vi "Minesweeper.vi"() -> ()   [LabVIEW 2018]
uses:
  ecc87c49-68d8-480b-962c-e2d9a9991d5a.vi
panel:
  in  "I did not survive and \nneed to try again:(":bool
  in  "Array":bool[][](array[boolean])
  out "Array 2":picture[][](array[picture])
  # "MINESWEEPER"
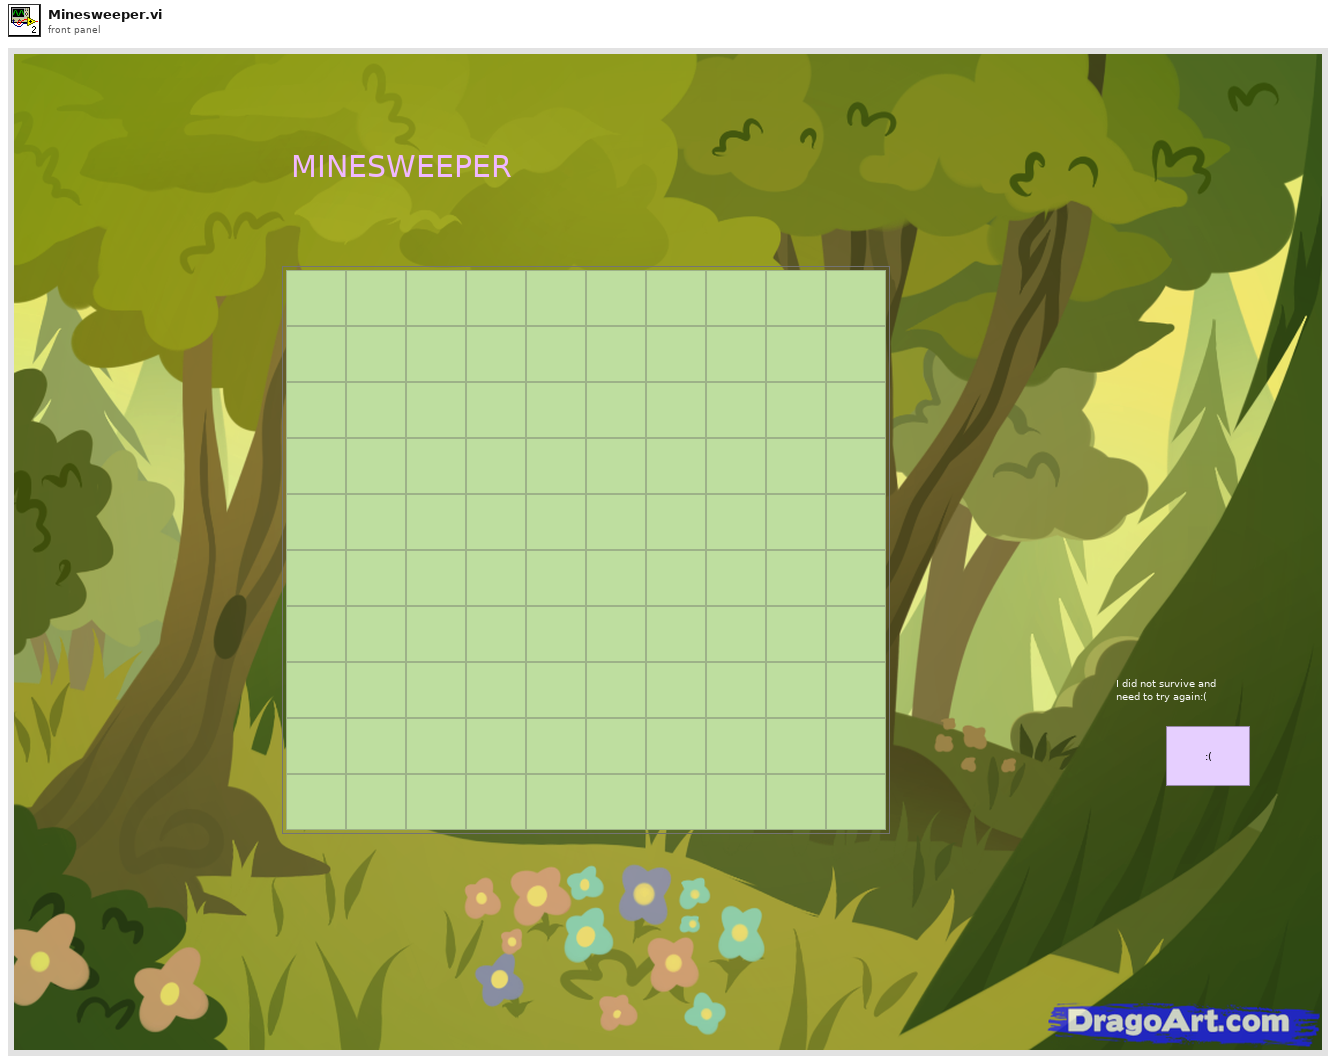
[diagram p1: front panel]
types:
  T1 = enum16{"Initialize", "Wait for event", "Game", "Analyze", "User msg", "New", "End"}
  T2 = typedef "imagedata.ctl" = cluster{"image type":i32, "image depth":i32, "image":u8[], "mask":u8[], "colors":u32[], "Rectangle":cluster{"left":i16, "top":i16, "right":i16, "bottom":i16}}
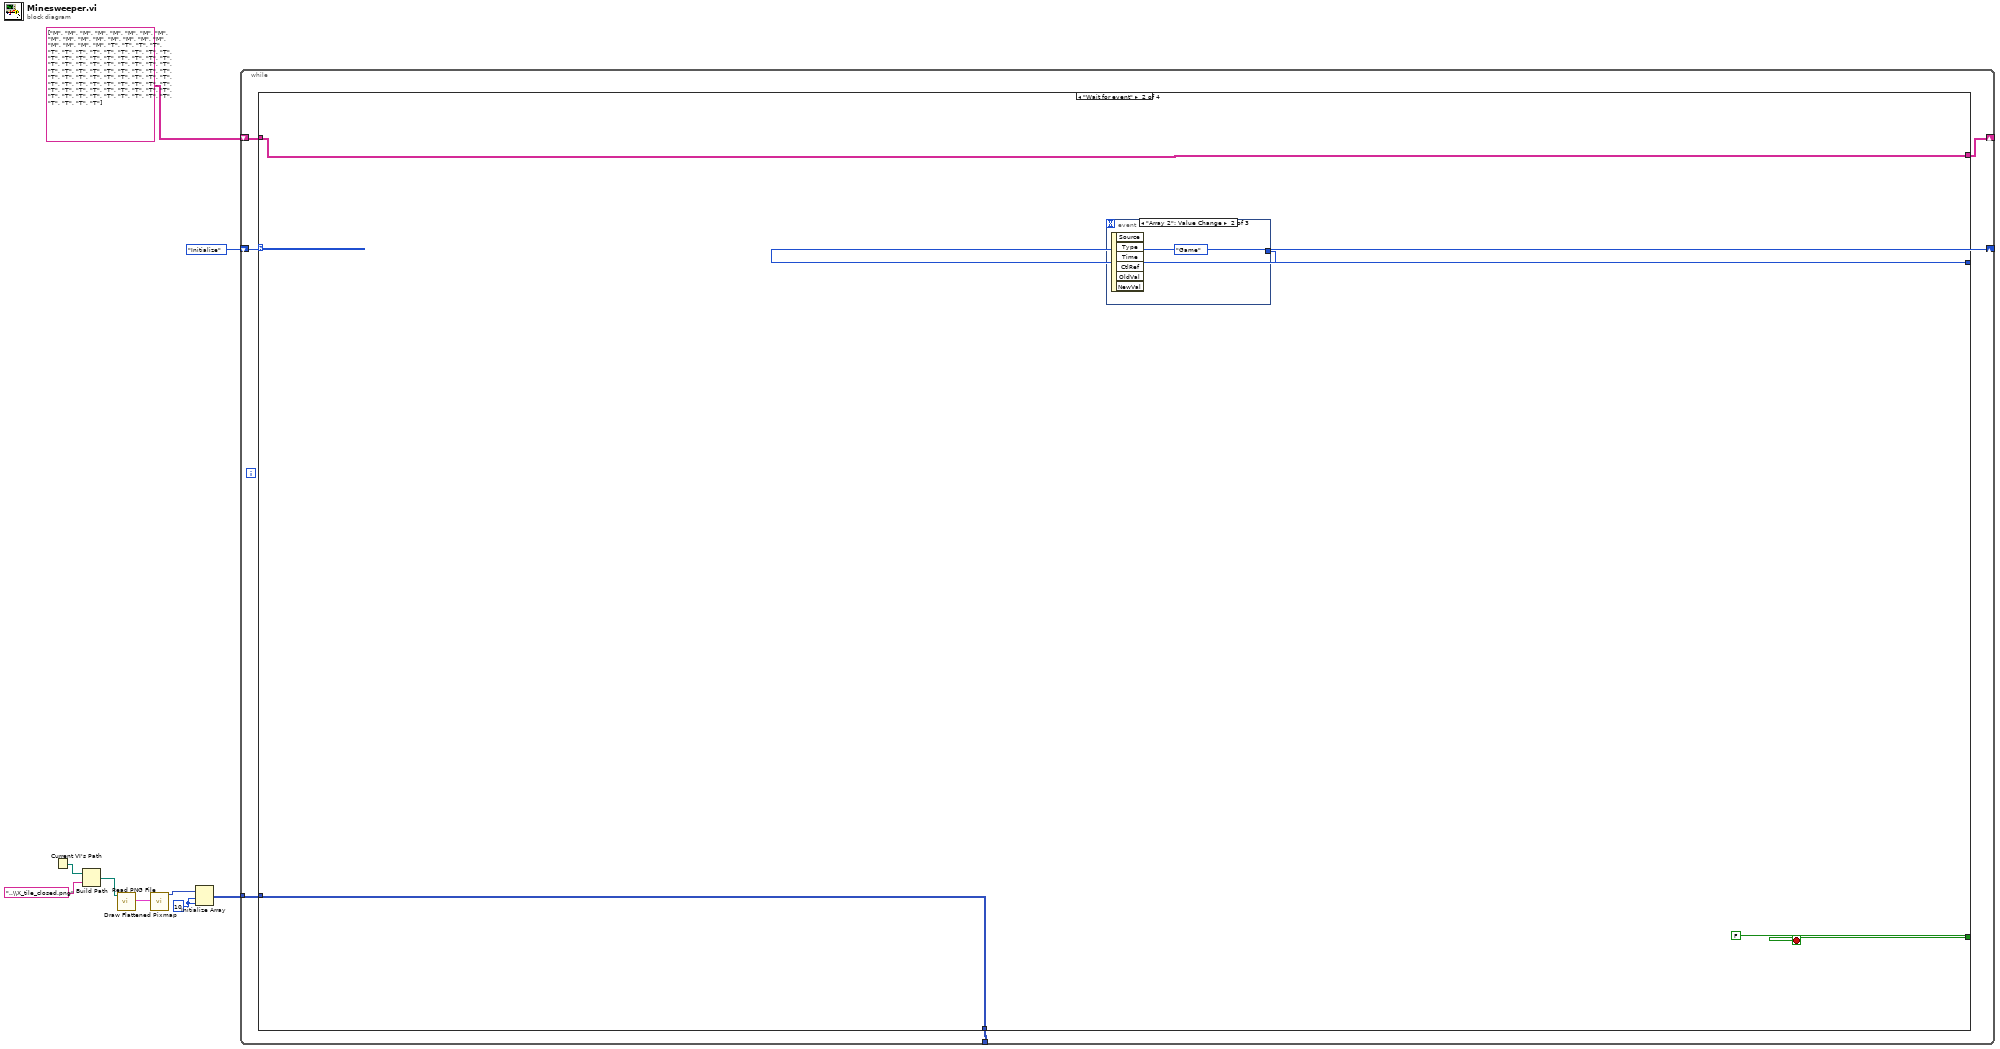
[diagram p0: block diagram]
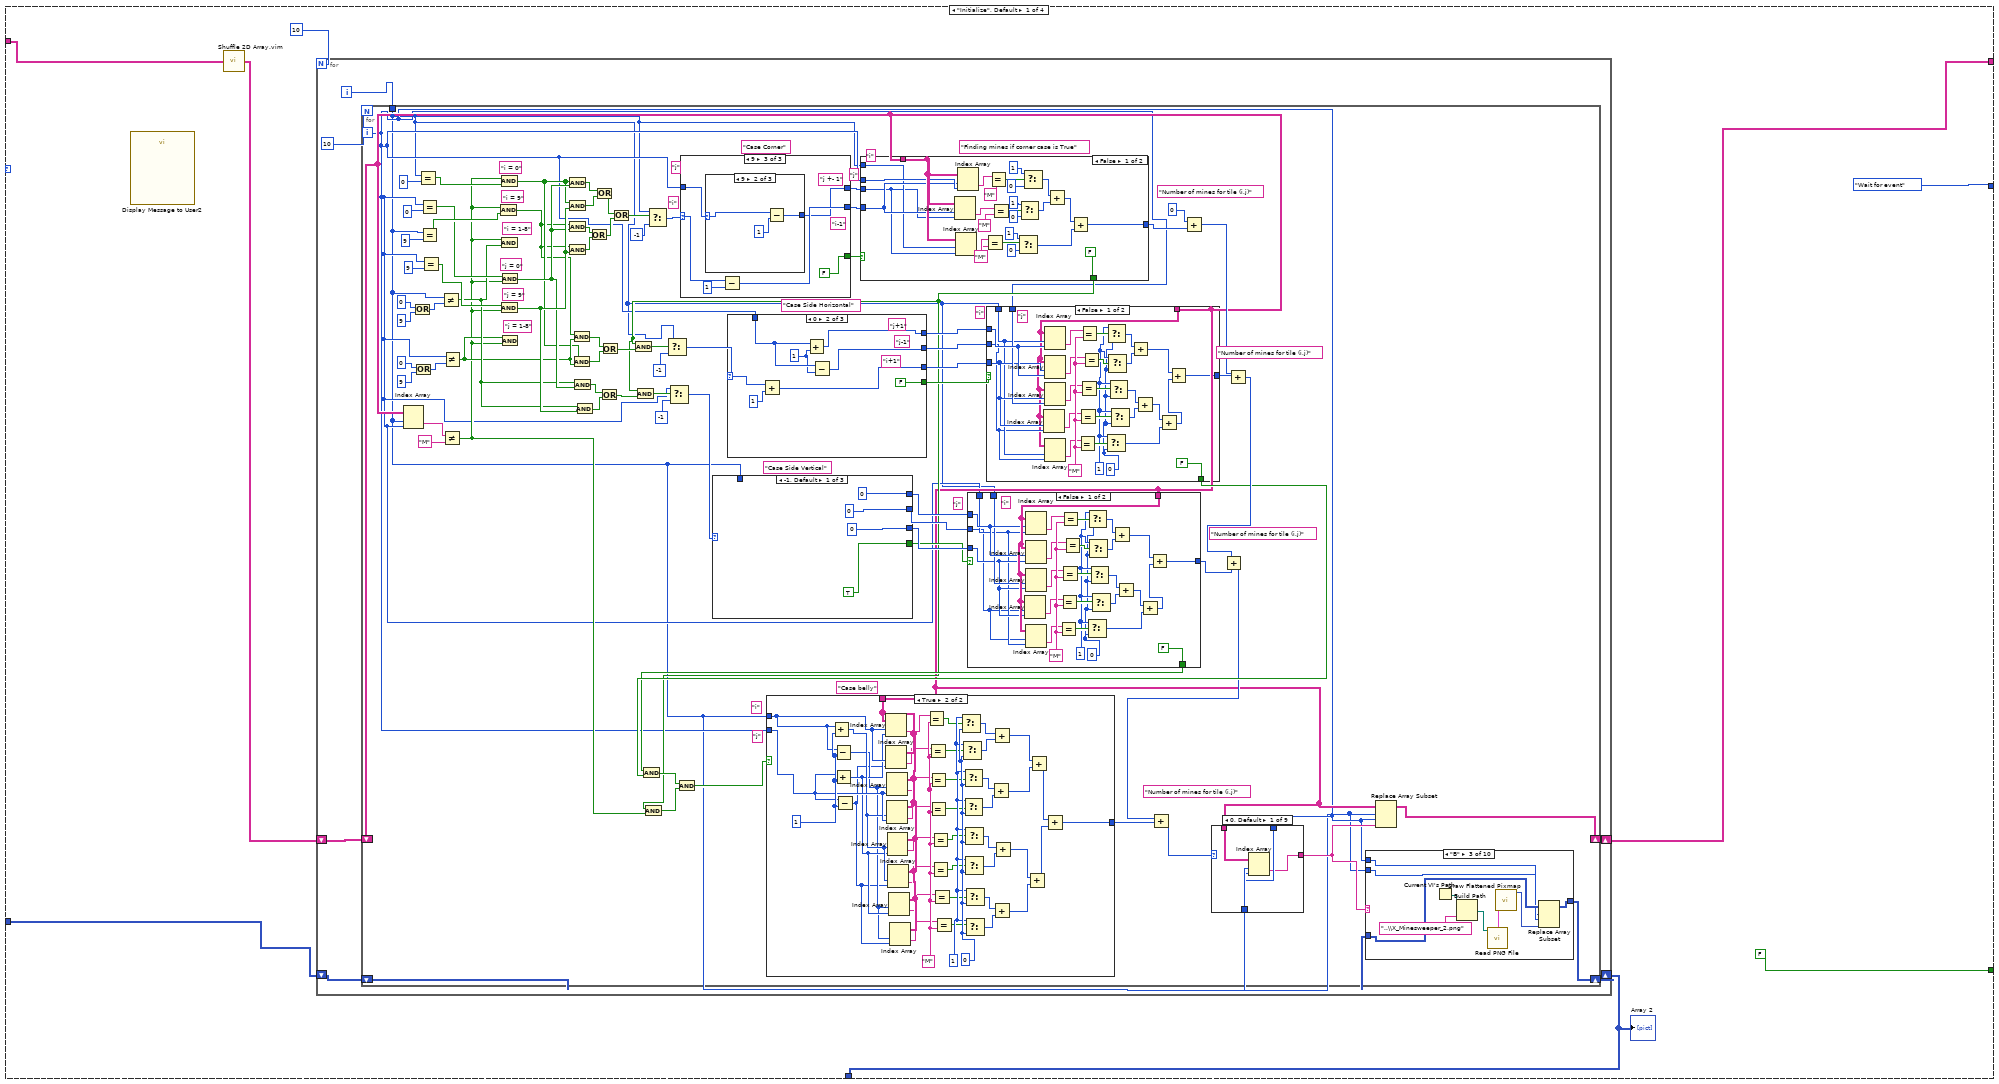
[diagram p2: hidden frame]
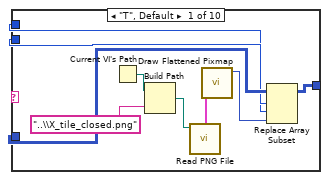
[diagram p3: hidden frame]
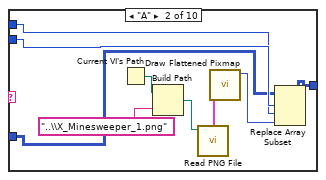
[diagram p4: hidden frame]
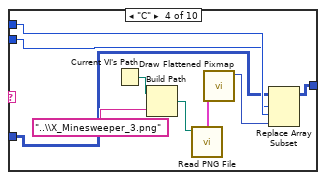
[diagram p5: hidden frame]
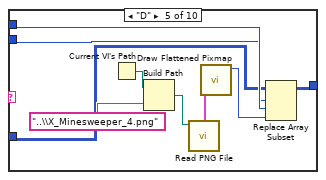
[diagram p6: hidden frame]
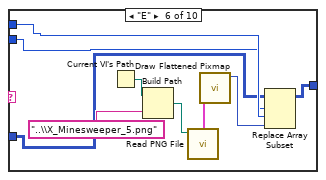
[diagram p7: hidden frame]
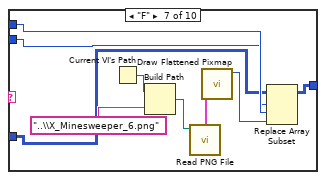
[diagram p8: hidden frame]
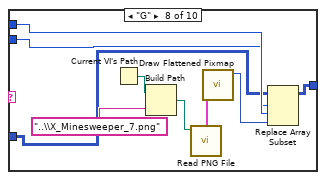
[diagram p9: hidden frame]
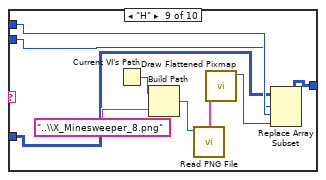
[diagram p10: hidden frame]
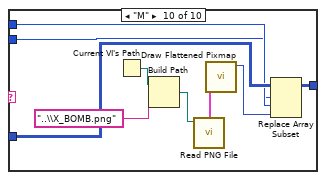
[diagram p11: hidden frame]
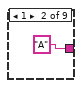
[diagram p12: hidden frame]
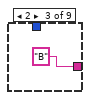
[diagram p13: hidden frame]
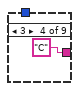
[diagram p14: hidden frame]
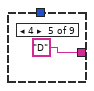
[diagram p15: hidden frame]
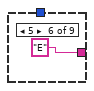
[diagram p16: hidden frame]
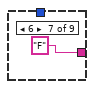
[diagram p17: hidden frame]
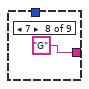
[diagram p18: hidden frame]
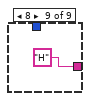
[diagram p19: hidden frame]
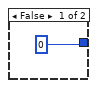
[diagram p20: hidden frame]
diagram:
  w2 = 10
  n1 = Current VI's Path() -> (path=w4:path)
  n2 = Build Path(base path=w4, name or relative path="..\\X_tile_closed.png") -> (appended path=w5:path)
  n3 = call <vilib>:"Read PNG File.vi"("path to PNG file"=w5) -> ("image data"=w6:T2)  [unwired: 8 in, 2 out]
  n4 = call <vilib>:"Draw Flattened Pixmap.vi"("image data"=w6) -> ("new picture"=w7:picture)  [unwired: 8 in]
  n5 = Initialize Array(w7, w2, w2) -> (w1:picture[][])
  n6 = while {
    shift-right: [w15] -> _
    shift-left: T1."Initialize" -> [w16]
    tunnel: w1 -> [w13]
    tunnel: [w12] -> _
    shift-right: [w10] -> _
    shift-left: string[][] [["M", "M", "M", "M", "M", "M", "M", "M", "M", "M"], ["M", "M", "M", "M", "M", "M", "M", "M", "M", "M"], ["T", "T", "T", "T", "T", "T", "T", "T", "T", "T"], ["T", "T", "T", "T", "T", "T", "T", "T", "T", "T"], ["T", "T", "T", "T", "T", "T", "T", "T", "T", "T"], ["T", "T", "T", "T", "T", "T", "T", "T", "T", "T"], ["T", "T", "T", "T", "T", "T", "T", "T", "T", "T"], ["T", "T", "T", "T", "T", "T", "T", "T", "T", "T"], ["T", "T", "T", "T", "T", "T", "T", "T", "T", "T"], ["T", "T", "T", "T", "T", "T", "T", "T", "T", "T"]] -> [w11]
    stop <- w14 stop-if-true
    n7 = case shown="\"Wait for event\"" w16 {
      tunnel: [w20 w416 w429 string[][] [["M", "M", "M", "M", "M", "M", "M", "M", "M", "M"], ["M", "M", "M", "M", "M", "M", "M", "M", "M", "M"], ["T", "T", "T", "T", "T", "T", "T", "T", "T", "T"], ["T", "T", "T", "T", "T", "T", "T", "T", "T", "T"], ["T", "T", "T", "T", "T", "T", "T", "T", "T", "T"], ["T", "T", "T", "T", "T", "T", "T", "T", "T", "T"], ["T", "T", "T", "T", "T", "T", "T", "T", "T", "T"], ["T", "T", "T", "T", "T", "T", "T", "T", "T", "T"], ["T", "T", "T", "T", "T", "T", "T", "T", "T", "T"], ["T", "T", "T", "T", "T", "T", "T", "T", "T", "T"]]] -> w10
      tunnel: [T1."Wait for event" w417 T1."Wait for event" T1."Initialize"] -> w15
      tunnel: [FALSE FALSE FALSE FALSE] -> w14
      tunnel: [w19 w415 w427 w457] -> w12
      tunnel: w13 -> [w18 w415 w427 w457]
      tunnel: w11 -> [w17 w416 w429 _]
      frame "Initialize", Default {
        n8 = call "Display Message to User2"() -> ()  [unwired: 10 in, 2 out]
        n9 = call "Shuffle 2D Array.vim"("array"=w17) -> ("shuffled array"=w21:string[][])  [unwired: 4 in]
        n10 = for {
          N: 10 -> [_]
          shift-right: [w28] -> w20
          shift-left: w21 -> [w29]
          shift-right: [w25] -> w19
          shift-left: w18 -> [w26]
          i -> [w27]
          n11 = for {
            N: 10 -> [_]
            tunnel: w27 -> [w32]
            shift-right: [w45] -> w28
            shift-left: w29 -> [w36]
            shift-right: [w31] -> w25
            shift-left: w26 -> [w34]
            i -> [w33]
            (unwired) "j"
            (unwired) "i"
            (unwired) "j"
            (unwired) "i"
            (unwired) "j"
            (unwired) "Number of mines for tile (i,j)"
            (unwired) "j"
            (unwired) "i"
            (unwired) "Case belly"
            (unwired) "Case Side Vertical"
            (unwired) "Number of mines for tile (i,j)"
            (unwired) "Number of mines for tile (i,j)"
            (unwired) "i"
            (unwired) "Case Side Horizontal"
            (unwired) "Finding mines if corner case is True"
            (unwired) "Number of mines for tile (i,j)"
            (unwired) "Case Corner"
            (unwired) "j = 1-8"
            (unwired) "j = 9"
            (unwired) "j = 0"
            (unwired) "i = 1-8"
            (unwired) "i = 9"
            (unwired) "i = 0"
            n12 = Index Array(array=w36, index (row)=w32, index (col)=w33) -> (element=w106:string)
            n13 = Or(x=0, y=9) -> (x .or. y?=w37:i32)
            n14 = Or(x=0, y=9) -> (x .or. y?=w99:i32)
            n15 = Equal?(x=w32, y=0) -> (x = y?=w98:bool)
            n16 = Equal?(x=w33, y=0) -> (x = y?=w96:bool)
            n17 = Equal?(x=w32, y=9) -> (x = y?=w97:bool)
            n18 = Equal?(x=w33, y=9) -> (x = y?=w95:bool)
            n19 = Not Equal?(x=w32, y=w37) -> (x != y?=w78:bool)
            n20 = Not Equal?(x=w106, y="M") -> (x != y?=w41:bool)
            n21 = Not Equal?(x=w33, y=w99) -> (x != y?=w77:bool)
            n22 = And(x=w41, y=w97) -> (x .and. y?=w75:bool)
            n23 = And(x=w41, y=w98) -> (x .and. y?=w76:bool)
            n24 = And(x=w41, y=w78) -> ()  [unwired: 1 out]
            n25 = And(x=w95, y=w41) -> (x .and. y?=w80:bool)
            n26 = And(x=w96, y=w41) -> (x .and. y?=w79:bool)
            n27 = And(x=w77, y=w41) -> ()  [unwired: 1 out]
            n28 = And(x=w76, y=w79) -> (x .and. y?=w94:bool)
            n29 = And(x=w76, y=w80) -> (x .and. y?=w93:bool)
            n30 = And(x=w75, y=w79) -> (x .and. y?=w92:bool)
            n31 = And(x=w75, y=w80) -> (x .and. y?=w91:bool)
            n32 = And(x=w75, y=w77) -> (x .and. y?=w74:bool)
            n33 = And(x=w76, y=w77) -> (x .and. y?=w73:bool)
            n34 = And(x=w78, y=w79) -> (x .and. y?=w72:bool)
            n35 = And(x=w78, y=w80) -> (x .and. y?=w71:bool)
            n36 = Or(x=w92, y=w91) -> (x .or. y?=w89:bool)
            n37 = Or(x=w94, y=w93) -> (x .or. y?=w90:bool)
            n38 = Or(x=w72, y=w71) -> (x .or. y?=w64:bool)
            n39 = Or(x=w74, y=w73) -> (x .or. y?=w69:bool)
            n40 = Or(x=w90, y=w89) -> (x .or. y?=w88:bool)
            n41 = Select(t=w32, s=w88, f=-1) -> (s? t:f=w86:i32)
            n42 = case shown="9" w86 {
              selector: w86 -> [w384 w392 w404]
              tunnel: [TRUE FALSE FALSE] -> w85
              tunnel: [w383 w390 w403] -> w84
              tunnel: w33 -> [w386 w388 w401]
              tunnel: [w385 w389 w402] -> w83
              frame -1, Default {
                n43 = Subtract(x=w386, y=w386) -> (x-y=w385:i32)
                n44 = Subtract(x=w384, y=w384) -> (x-y=w383:i32)
              }
              frame 0 {
                (unwired) "j +- 1"
                (unwired) "i+1"
                n45 = case shown="-1, Default" w388 {
                  selector: w388 -> [w396 w397 w399]
                  tunnel: [w394 w397 w398] -> w389
                  frame 0 {
                    n46 = Add(x=w396, y=1) -> (x+y=w394:i32)
                  }
                  frame -1, Default {
                  }
                  frame 9 {
                    n47 = Subtract(x=w399, y=1) -> (x-y=w398:i32)
                  }
                }
                n48 = Add(x=w392, y=1) -> (x+y=w390:i32)
              }
              frame 9 {
                (unwired) "j +- 1"
                (unwired) "i-1"
                n49 = case shown="9" w401 {
                  selector: w401 -> [w409 w411 w413]
                  tunnel: [w407 w410 w413] -> w402
                  frame 0 {
                    n50 = Add(x=w409, y=1) -> (x+y=w407:i32)
                  }
                  frame 9 {
                    n51 = Subtract(x=w411, y=1) -> (x-y=w410:i32)
                  }
                  frame -1, Default {
                  }
                }
                n52 = Subtract(x=w404, y=1) -> (x-y=w403:i32)
              }
            }
            n53 = case shown="False" w85 {
              tunnel: [FALSE TRUE] -> w42
              tunnel: w84 -> [w377 _]
              tunnel: w83 -> [w375 _]
              tunnel: w33 -> [w378 _]
              tunnel: w32 -> [w376 _]
              tunnel: w36 -> [w379 _]
              tunnel: [w355 0] -> w81
              frame False {
                n54 = Index Array(array=w379, index (row)=w377, index (col)=w375) -> (element=w372:string)
                n55 = Index Array(array=w379, index (row)=w376, index (col)=w375) -> (element=w370:string)
                n56 = Index Array(array=w379, index (row)=w377, index (col)=w378) -> (element=w374:string)
                n57 = Equal?(x=w370, y="M") -> (x = y?=w366:bool)
                n58 = Equal?(x=w374, y="M") -> (x = y?=w368:bool)
                n59 = Equal?(x=w372, y="M") -> (x = y?=w367:bool)
                n60 = Select(t=1, s=w366, f=0) -> (s? t:f=w356:i32)
                n61 = Select(t=1, s=w367, f=0) -> (s? t:f=w358:i32)
                n62 = Select(t=1, s=w368, f=0) -> (s? t:f=w359:i32)
                n63 = Add(x=w359, y=w358) -> (x+y=w357:i32)
                n64 = Add(x=w357, y=w356) -> (x+y=w355:i32)
              }
              frame True {
              }
            }
            n65 = And(x=w42, y=w69) -> (x .and. y?=w68:bool)
            n66 = And(x=w42, y=w64) -> (x .and. y?=w65:bool)
            n67 = And(x=w42, y=w41) -> (x .and. y?=w40:bool)
            n68 = Select(t=w32, s=w68, f=-1) -> (s? t:f=w67:i32)
            n69 = Select(t=w33, s=w65, f=-1) -> (s? t:f=w63:i32)
            n70 = case shown="-1, Default" w63 {
              selector: w63 -> [_ w319 w328]
              tunnel: [TRUE FALSE FALSE] -> w47
              tunnel: [0 w325 w329] -> w54
              tunnel: [0 w320 w331] -> w55
              tunnel: w32 -> [_ w323 w333]
              tunnel: [0 w321 w332] -> w56
              frame -1, Default {
              }
              frame 0 {
                (unwired) "j+1"
                (unwired) "i-1"
                (unwired) "i+1"
                w322 = 1
                n71 = Add(x=w319, y=1) -> (x+y=w325:i32)
                n72 = Add(x=w323, y=w322) -> (x+y=w321:i32)
                n73 = Subtract(x=w323, y=w322) -> (x-y=w320:i32)
              }
              frame 9 {
                (unwired) "j-1"
                (unwired) "i-1"
                (unwired) "i+1"
                w334 = 1
                n74 = Subtract(x=w328, y=1) -> (x-y=w329:i32)
                n75 = Add(x=w333, y=w334) -> (x+y=w332:i32)
                n76 = Subtract(x=w333, y=w334) -> (x-y=w331:i32)
              }
            }
            n77 = case shown="0" w67 {
              selector: w67 -> [_ w345 w348]
              tunnel: [TRUE FALSE FALSE] -> w61
              tunnel: [0 w344 w349] -> w62
              tunnel: [0 w339 w351] -> w60
              tunnel: w33 -> [_ w342 w353]
              tunnel: [0 w340 w352] -> w59
              frame -1, Default {
              }
              frame 0 {
                (unwired) "i+1"
                (unwired) "j-1"
                (unwired) "j+1"
                w341 = 1
                n78 = Add(x=w345, y=1) -> (x+y=w344:i32)
                n79 = Add(x=w342, y=w341) -> (x+y=w340:i32)
                n80 = Subtract(x=w342, y=w341) -> (x-y=w339:i32)
              }
              frame 9 {
                (unwired) "i-1"
                (unwired) "j-1"
                (unwired) "j+1"
                w354 = 1
                n81 = Subtract(x=w348, y=1) -> (x-y=w349:i32)
                n82 = Add(x=w353, y=w354) -> (x+y=w352:i32)
                n83 = Subtract(x=w353, y=w354) -> (x-y=w351:i32)
              }
            }
            n84 = case shown="False" w47 {
              tunnel: w54 -> [w255 _]
              tunnel: w55 -> [w253 _]
              tunnel: w56 -> [w257 _]
              tunnel: w33 -> [w254 _]
              tunnel: w32 -> [w256 _]
              tunnel: w36 -> [w280 _]
              tunnel: [w259 0] -> w52
              tunnel: [FALSE TRUE] -> w50
              frame False {
                (unwired) "i"
                w268 = 0
                w269 = 1
                w281 = "M"
                n85 = Index Array(array=w280, index (row)=w253, index (col)=w255) -> (element=w276:string)
                n86 = Index Array(array=w280, index (row)=w257, index (col)=w254) -> (element=w279:string)
                n87 = Index Array(array=w280, index (row)=w257, index (col)=w255) -> (element=w278:string)
                n88 = Index Array(array=w280, index (row)=w256, index (col)=w255) -> (element=w277:string)
                n89 = Index Array(array=w280, index (row)=w253, index (col)=w254) -> (element=w275:string)
                n90 = Equal?(x=w275, y=w281) -> (x = y?=w270:bool)
                n91 = Equal?(x=w276, y=w281) -> (x = y?=w271:bool)
                n92 = Equal?(x=w277, y=w281) -> (x = y?=w272:bool)
                n93 = Equal?(x=w279, y=w281) -> (x = y?=w274:bool)
                n94 = Equal?(x=w278, y=w281) -> (x = y?=w273:bool)
                n95 = Select(t=w269, s=w270, f=w268) -> (s? t:f=w263:i32)
                n96 = Select(t=w269, s=w274, f=w268) -> (s? t:f=w264:i32)
                n97 = Select(t=w269, s=w273, f=w268) -> (s? t:f=w265:i32)
                n98 = Select(t=w269, s=w272, f=w268) -> (s? t:f=w266:i32)
                n99 = Select(t=w269, s=w271, f=w268) -> (s? t:f=w267:i32)
                n100 = Add(x=w264, y=w265) -> (x+y=w260:i32)
                n101 = Add(x=w266, y=w267) -> (x+y=w262:i32)
                n102 = Add(x=w262, y=w263) -> (x+y=w261:i32)
                n103 = Add(x=w260, y=w261) -> (x+y=w259:i32)
              }
              frame True {
              }
            }
            n104 = case shown="False" w61 {
              tunnel: w62 -> [w310 _]
              tunnel: w60 -> [w308 _]
              tunnel: w59 -> [w312 _]
              tunnel: w32 -> [w309 _]
              tunnel: w33 -> [w311 _]
              tunnel: w36 -> [w306 _]
              tunnel: [w285 0] -> w57
              tunnel: [FALSE TRUE] -> w51
              frame False {
                (unwired) "j"
                w294 = 0
                w295 = 1
                w307 = "M"
                n105 = Index Array(array=w306, index (row)=w310, index (col)=w308) -> (element=w302:string)
                n106 = Index Array(array=w306, index (row)=w309, index (col)=w312) -> (element=w305:string)
                n107 = Index Array(array=w306, index (row)=w310, index (col)=w312) -> (element=w304:string)
                n108 = Index Array(array=w306, index (row)=w310, index (col)=w311) -> (element=w303:string)
                n109 = Index Array(array=w306, index (row)=w309, index (col)=w308) -> (element=w301:string)
                n110 = Equal?(x=w301, y=w307) -> (x = y?=w296:bool)
                n111 = Equal?(x=w302, y=w307) -> (x = y?=w297:bool)
                n112 = Equal?(x=w303, y=w307) -> (x = y?=w298:bool)
                n113 = Equal?(x=w305, y=w307) -> (x = y?=w300:bool)
                n114 = Equal?(x=w304, y=w307) -> (x = y?=w299:bool)
                n115 = Select(t=w295, s=w296, f=w294) -> (s? t:f=w289:i32)
                n116 = Select(t=w295, s=w300, f=w294) -> (s? t:f=w290:i32)
                n117 = Select(t=w295, s=w299, f=w294) -> (s? t:f=w291:i32)
                n118 = Select(t=w295, s=w298, f=w294) -> (s? t:f=w292:i32)
                n119 = Select(t=w295, s=w297, f=w294) -> (s? t:f=w293:i32)
                n120 = Add(x=w290, y=w291) -> (x+y=w286:i32)
                n121 = Add(x=w292, y=w293) -> (x+y=w288:i32)
                n122 = Add(x=w288, y=w289) -> (x+y=w287:i32)
                n123 = Add(x=w286, y=w287) -> (x+y=w285:i32)
              }
              frame True {
                (unwired) "j"
              }
            }
            n124 = And(x=w50, y=w51) -> (x .and. y?=w44:bool)
            n125 = And(x=w44, y=w40) -> (x .and. y?=w43:bool)
            n126 = case shown="True" w43 {
              tunnel: w32 -> [_ w216]
              tunnel: w33 -> [_ w215]
              tunnel: w36 -> [_ w250]
              tunnel: [0 w217] -> w48
              frame False {
              }
              frame True {
                w241 = 0
                w240 = 1
                w251 = "M"
                w252 = 1
                n127 = Add(x=w216, y=w252) -> (x+y=w214:i32)
                n128 = Subtract(x=w216, y=w252) -> (x-y=w212:i32)
                n129 = Add(x=w215, y=w252) -> (x+y=w213:i32)
                n130 = Subtract(x=w215, y=w252) -> (x-y=w211:i32)
                n131 = Index Array(array=w250, index (row)=w216, index (col)=w213) -> (element=w242:string)
                n132 = Index Array(array=w250, index (row)=w216, index (col)=w211) -> (element=w243:string)
                n133 = Index Array(array=w250, index (row)=w212, index (col)=w215) -> (element=w244:string)
                n134 = Index Array(array=w250, index (row)=w214, index (col)=w215) -> (element=w245:string)
                n135 = Index Array(array=w250, index (row)=w214, index (col)=w213) -> (element=w246:string)
                n136 = Index Array(array=w250, index (row)=w214, index (col)=w211) -> (element=w247:string)
                n137 = Index Array(array=w250, index (row)=w212, index (col)=w213) -> (element=w248:string)
                n138 = Index Array(array=w250, index (row)=w212, index (col)=w211) -> (element=w249:string)
                n139 = Equal?(x=w242, y=w251) -> (x = y?=w239:bool)
                n140 = Equal?(x=w243, y=w251) -> (x = y?=w238:bool)
                n141 = Equal?(x=w244, y=w251) -> (x = y?=w237:bool)
                n142 = Equal?(x=w245, y=w251) -> (x = y?=w236:bool)
                n143 = Equal?(x=w246, y=w251) -> (x = y?=w235:bool)
                n144 = Equal?(x=w247, y=w251) -> (x = y?=w234:bool)
                n145 = Equal?(x=w248, y=w251) -> (x = y?=w233:bool)
                n146 = Equal?(x=w249, y=w251) -> (x = y?=w232:bool)
                n147 = Select(t=w240, s=w239, f=w241) -> (s? t:f=w224:i32)
                n148 = Select(t=w240, s=w238, f=w241) -> (s? t:f=w225:i32)
                n149 = Select(t=w240, s=w237, f=w241) -> (s? t:f=w226:i32)
                n150 = Select(t=w240, s=w236, f=w241) -> (s? t:f=w227:i32)
                n151 = Select(t=w240, s=w235, f=w241) -> (s? t:f=w228:i32)
                n152 = Select(t=w240, s=w234, f=w241) -> (s? t:f=w229:i32)
                n153 = Select(t=w240, s=w233, f=w241) -> (s? t:f=w230:i32)
                n154 = Select(t=w240, s=w232, f=w241) -> (s? t:f=w231:i32)
                n155 = Add(x=w226, y=w227) -> (x+y=w222:i32)
                n156 = Add(x=w224, y=w225) -> (x+y=w223:i32)
                n157 = Add(x=w230, y=w231) -> (x+y=w220:i32)
                n158 = Add(x=w228, y=w229) -> (x+y=w221:i32)
                n159 = Add(x=w221, y=w220) -> (x+y=w219:i32)
                n160 = Add(x=w223, y=w222) -> (x+y=w218:i32)
                n161 = Add(x=w218, y=w219) -> (x+y=w217:i32)
              }
            }
            n162 = Add(x=0, y=w81) -> (x+y=w58:i32)
            n163 = Add(x=w58, y=w57) -> (x+y=w53:i32)
            n164 = Add(x=w53, y=w52) -> (x+y=w49:i32)
            n165 = Add(x=w49, y=w48) -> (x+y=w46:i32)
            n166 = case shown="0, Default" w46 {
              tunnel: [w198 "A" "B" "C" "D" "E" "F" "G" "H"] -> w35
              tunnel: w36 -> [w201 _ _ _ _ _ _ _ _]
              tunnel: w32 -> [w200 _ _ _ _ _ _ _ _]
              tunnel: w33 -> [w199 _ _ _ _ _ _ _ _]
              frame 0, Default {
                n167 = Index Array(array=w201, index (row)=w200, index (col)=w199) -> (element=w198:string)
              }
              frame 1 {
              }
              frame 2 {
              }
              frame 3 {
              }
              frame 4 {
              }
              frame 5 {
              }
              frame 6 {
              }
              frame 7 {
              }
              frame 8 {
              }
            }
            n168 = case shown="\"B\"" w35 {
              tunnel: w34 -> [w111 w118 w129 w136 w145 w154 w163 w172 w181 w193]
              tunnel: w33 -> [w109 w119 w128 w138 w147 w156 w165 w174 w183 w192]
              tunnel: w32 -> [w110 w120 w127 w137 w146 w155 w164 w173 w182 w191]
              tunnel: [w108 w117 w126 w135 w144 w153 w162 w171 w180 w189] -> w31
              frame "T", Default {
                n169 = Current VI's Path() -> (path=w115:path)
                n170 = Build Path(base path=w115, name or relative path="..\\X_tile_closed.png") -> (appended path=w114:path)
                n171 = call <vilib>:"Read PNG File.vi"("path to PNG file"=w114) -> ("image data"=w113:T2)  [unwired: 8 in, 2 out]
                n172 = call <vilib>:"Draw Flattened Pixmap.vi"("image data"=w113) -> ("new picture"=w116:picture)  [unwired: 8 in]
                n173 = Replace Array Subset(array=w111, new element=w116, index (row)=w110, index (col)=w109) -> (w108:picture[][])
              }
              frame "A" {
                n174 = Current VI's Path() -> (path=w124:path)
                n175 = Build Path(base path=w124, name or relative path="..\\X_Minesweeper_1.png") -> (appended path=w123:path)
                n176 = call <vilib>:"Read PNG File.vi"("path to PNG file"=w123) -> ("image data"=w122:T2)  [unwired: 8 in, 2 out]
                n177 = call <vilib>:"Draw Flattened Pixmap.vi"("image data"=w122) -> ("new picture"=w125:picture)  [unwired: 8 in]
                n178 = Replace Array Subset(array=w118, new element=w125, index (row)=w120, index (col)=w119) -> (w117:picture[][])
              }
              frame "B" {
                n179 = Current VI's Path() -> (path=w133:path)
                n180 = Build Path(base path=w133, name or relative path="..\\X_Minesweeper_2.png") -> (appended path=w132:path)
                n181 = call <vilib>:"Read PNG File.vi"("path to PNG file"=w132) -> ("image data"=w131:T2)  [unwired: 8 in, 2 out]
                n182 = call <vilib>:"Draw Flattened Pixmap.vi"("image data"=w131) -> ("new picture"=w134:picture)  [unwired: 8 in]
                n183 = Replace Array Subset(array=w129, new element=w134, index (row)=w127, index (col)=w128) -> (w126:picture[][])
              }
              frame "C" {
                n184 = Current VI's Path() -> (path=w141:path)
                n185 = Build Path(base path=w141, name or relative path="..\\X_Minesweeper_3.png") -> (appended path=w142:path)
                n186 = call <vilib>:"Read PNG File.vi"("path to PNG file"=w142) -> ("image data"=w143:T2)  [unwired: 8 in, 2 out]
                n187 = call <vilib>:"Draw Flattened Pixmap.vi"("image data"=w143) -> ("new picture"=w140:picture)  [unwired: 8 in]
                n188 = Replace Array Subset(array=w136, new element=w140, index (row)=w137, index (col)=w138) -> (w135:picture[][])
              }
              frame "D" {
                n189 = Current VI's Path() -> (path=w150:path)
                n190 = Build Path(base path=w150, name or relative path="..\\X_Minesweeper_4.png") -> (appended path=w151:path)
                n191 = call <vilib>:"Read PNG File.vi"("path to PNG file"=w151) -> ("image data"=w152:T2)  [unwired: 8 in, 2 out]
                n192 = call <vilib>:"Draw Flattened Pixmap.vi"("image data"=w152) -> ("new picture"=w149:picture)  [unwired: 8 in]
                n193 = Replace Array Subset(array=w145, new element=w149, index (row)=w146, index (col)=w147) -> (w144:picture[][])
              }
              frame "E" {
                n194 = Current VI's Path() -> (path=w159:path)
                n195 = Build Path(base path=w159, name or relative path="..\\X_Minesweeper_5.png") -> (appended path=w160:path)
                n196 = call <vilib>:"Read PNG File.vi"("path to PNG file"=w160) -> ("image data"=w161:T2)  [unwired: 8 in, 2 out]
                n197 = call <vilib>:"Draw Flattened Pixmap.vi"("image data"=w161) -> ("new picture"=w158:picture)  [unwired: 8 in]
                n198 = Replace Array Subset(array=w154, new element=w158, index (row)=w155, index (col)=w156) -> (w153:picture[][])
              }
              frame "F" {
                n199 = Current VI's Path() -> (path=w168:path)
                n200 = Build Path(base path=w168, name or relative path="..\\X_Minesweeper_6.png") -> (appended path=w169:path)
                n201 = call <vilib>:"Read PNG File.vi"("path to PNG file"=w169) -> ("image data"=w170:T2)  [unwired: 8 in, 2 out]
                n202 = call <vilib>:"Draw Flattened Pixmap.vi"("image data"=w170) -> ("new picture"=w167:picture)  [unwired: 8 in]
                n203 = Replace Array Subset(array=w163, new element=w167, index (row)=w164, index (col)=w165) -> (w162:picture[][])
              }
              frame "G" {
                n204 = Current VI's Path() -> (path=w177:path)
                n205 = Build Path(base path=w177, name or relative path="..\\X_Minesweeper_7.png") -> (appended path=w178:path)
                n206 = call <vilib>:"Read PNG File.vi"("path to PNG file"=w178) -> ("image data"=w179:T2)  [unwired: 8 in, 2 out]
                n207 = call <vilib>:"Draw Flattened Pixmap.vi"("image data"=w179) -> ("new picture"=w176:picture)  [unwired: 8 in]
                n208 = Replace Array Subset(array=w172, new element=w176, index (row)=w173, index (col)=w174) -> (w171:picture[][])
              }
              frame "H" {
                n209 = Current VI's Path() -> (path=w186:path)
                n210 = Build Path(base path=w186, name or relative path="..\\X_Minesweeper_8.png") -> (appended path=w187:path)
                n211 = call <vilib>:"Read PNG File.vi"("path to PNG file"=w187) -> ("image data"=w188:T2)  [unwired: 8 in, 2 out]
                n212 = call <vilib>:"Draw Flattened Pixmap.vi"("image data"=w188) -> ("new picture"=w185:picture)  [unwired: 8 in]
                n213 = Replace Array Subset(array=w181, new element=w185, index (row)=w182, index (col)=w183) -> (w180:picture[][])
              }
              frame "M" {
                n214 = Current VI's Path() -> (path=w195:path)
                n215 = Build Path(base path=w195, name or relative path="..\\X_BOMB.png") -> (appended path=w196:path)
                n216 = call <vilib>:"Read PNG File.vi"("path to PNG file"=w196) -> ("image data"=w197:T2)  [unwired: 8 in, 2 out]
                n217 = call <vilib>:"Draw Flattened Pixmap.vi"("image data"=w197) -> ("new picture"=w190:picture)  [unwired: 8 in]
                n218 = Replace Array Subset(array=w193, new element=w190, index (row)=w191, index (col)=w192) -> (w189:picture[][])
              }
            }
            n219 = Replace Array Subset(array=w36, new element=w35, index (row)=w32, index (col)=w33) -> (w45:string[][])
          }
        }
        "Array 2" <- w19
      }
      frame "Wait for event" {
        n220 = event shown="[1] \"Array 2\": Value Change" {
          selector: _ -> [_ _ _]
          dyn-events: _ -> [_ _ _]
          timeout: _ -> [_ _ _]
          tunnel: [T1."New" T1."Game" T1."Game"] -> w417
          event "I did not survive and \nneed to try again:(": Value Change {
            n221 = event-data() -> ()  [unwired: 1 in, 6 out]
          }
          event "Array 2": Value Change {
            n222 = event-data() -> ()  [unwired: 1 in, 6 out]
          }
          event "Array": Value Change {
            n223 = event-data() -> ()  [unwired: 1 in, 6 out]
          }
        }
      }
      frame "Game" {
        w428 = 10
        n224 = for {
          N: w428 -> [_]
          tunnel: "Array" -> [w436]
          tunnel: w429 -> [w435]
          tunnel: w428 -> [w433]
          shift-right: [w431] -> w422
          shift-left: 0 -> [w432]
          i -> [w434]
          n225 = for {
            N: w433 -> [_]
            tunnel: w436 -> [w449]
            tunnel: w435 -> [w448]
            tunnel: w434 -> [w447]
            shift-right: [w437] -> w431
            shift-left: w432 -> [w438]
            i -> [w446]
            n226 = Index Array(array=w449, index (row)=w447, index (col)=w446) -> (element=w443:bool)
            n227 = Index Array(array=w448, index (row)=w447, index (col)=w446) -> (element=w445:string)
            n228 = Equal?(x=w443, y=TRUE) -> (x = y?=w439:bool)
            n229 = Equal?(x=w445, y="M") -> (x = y?=w441:bool)
            n230 = case shown="True" w439 {
              tunnel: w438 -> [w450 w453]
              tunnel: [w450 w451] -> w437
              frame False {
              }
              frame True {
                n231 = Add(x=w453, y=1) -> (x+y=w451:i32)
              }
            }
            n232 = And(x=w441, y=w439) -> (x .and. y?=w440:bool)
            n233 = case shown="True" w440 {
              frame False {
              }
              frame True {
                n234 = call "Display Message to User"("Message"="KABOOM! You lost:)" ("string")) -> ()  [unwired: 9 in, 2 out]
              }
            }
          }
        }
        n235 = Equal?(x=w422, y=80) -> (x = y?=w421:bool)
        n236 = case shown="True" w421 {
          frame False {
          }
          frame True {
            n237 = call "Display Message to User3"() -> ()  [unwired: 10 in, 2 out]
          }
        }
      }
      frame "New" {
        n238 = local write "Array"(bool[][] [[FALSE, FALSE, FALSE, FALSE, FALSE, FALSE, FALSE, FALSE, FALSE, FALSE], [FALSE, FALSE, FALSE, FALSE, FALSE, FALSE, FALSE, FALSE, FALSE, FALSE], [FALSE, FALSE, FALSE, FALSE, FALSE, FALSE, FALSE, FALSE, FALSE, FALSE], [FALSE, FALSE, FALSE, FALSE, FALSE, FALSE, FALSE, FALSE, FALSE, FALSE], [FALSE, FALSE, FALSE, FALSE, FALSE, FALSE, FALSE, FALSE, FALSE, FALSE], [FALSE, FALSE, FALSE, FALSE, FALSE, FALSE, FALSE, FALSE, FALSE, FALSE], [FALSE, FALSE, FALSE, FALSE, FALSE, FALSE, FALSE, FALSE, FALSE, FALSE], [FALSE, FALSE, FALSE, FALSE, FALSE, FALSE, FALSE, FALSE, FALSE, FALSE], [FALSE, FALSE, FALSE, FALSE, FALSE, FALSE, FALSE, FALSE, FALSE, FALSE], [FALSE, FALSE, FALSE, FALSE, FALSE, FALSE, FALSE, FALSE, FALSE, FALSE]]) -> ()
      }
    }
  }
